vi "Polish Control.vi"(10 "Control Ref":refnum<vi>, 11 "Array Writer in":refnum<class "Array Writer.lvclass">) -> (3 "Array Writer out":refnum<class "Array Writer.lvclass">)   [LabVIEW 2013, in "Array Writer.lvclass"]
doc: "Copyright (c) 2016 Sze Howe Koh\n\nThis Source Code Form is subject to the terms of the Mozilla Public License, v. 2.0. If a copy of the MPL was not distributed with this file, You can obtain one at http://mozilla.org/MPL/2.0/."
uses:
  Array Writer.lvclass
  Array Writer.lvclass/Array Writer.ctl
  Abstract Param Writer/Abstract Param Writer.lvclass
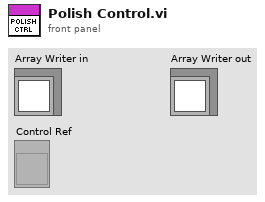
[diagram p1: front panel]
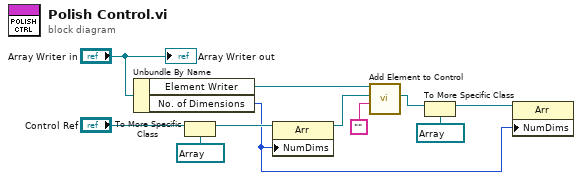
[diagram p0: block diagram]
diagram:
  n1 = Unbundle By Name("Array Writer in") -> ("Element Writer"=w11:refnum<class "Abstract Param Writer.lvclass">, "No. of Dimensions"=w1:u32)
  n2 = To More Specific Class(target class=refnum<vi> refnum ("Control Ref"), reference="Control Ref") -> (specific class reference=w6:refnum<vi>)  [unwired: 1 in, 1 out]
  n3 = property class="Arr"(reference=w6, "NumDims"=w1) -> (reference out=w5:refnum<vi>)  [unwired: 1 in, 1 out]
  n4 = call-dynamic "Add Element to Control.vi"("Element Name"="", "Cluster or Array"=w5, "Abstract Param Writer in"=w11) -> ("Cluster or Array Dup"=w2:refnum<vi>)  [unwired: 7 in, 1 out]
  n5 = To More Specific Class(target class=refnum<vi> refnum ("Control Ref"), reference=w2) -> (specific class reference=w4:refnum<vi>)  [unwired: 1 in, 1 out]
  n6 = property class="Arr"(reference=w4, "NumDims"=w1) -> ()  [unwired: 1 in, 2 out]
  "Array Writer out" <- "Array Writer in"
